vi "Swap_Joysticks.vi"(5 "Hold Time(ms)":u32, 6 "Axes 1 In":T1, 7 "Joystick 1":T2, 8 "Axes 0 in":T1, 9 "Joystick 0":T2) -> (0 "Axes 1 out":T1, 1 "Joystick 1 out":T2, 2 "Axes 0 out":T1, 3 "Joystick 0 Out":T2, 4 "Swap?":bool)   [LabVIEW 2017]
uses:
  ArgosLib/Signal Processing/TypeDefs/EdgeDetector_Type.ctl
  ArgosLib/ArgosLib.lvlib
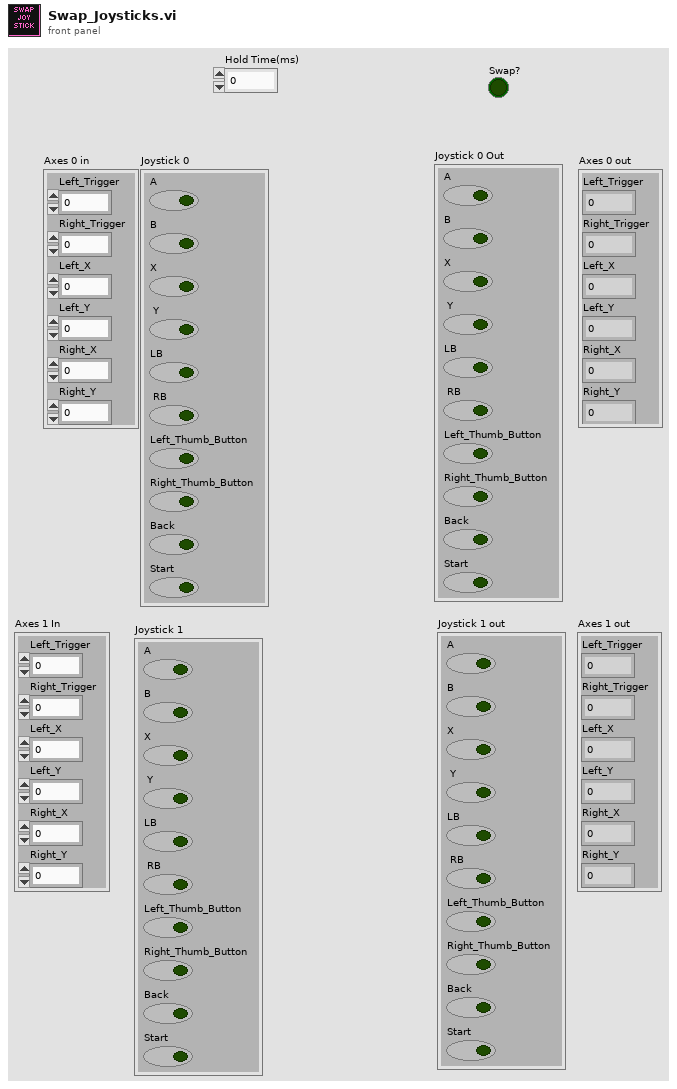
[diagram p1: front panel]
types:
  T1 = cluster{"Left_Trigger":dbl, "Right_Trigger ":dbl, "Left_X":dbl, "Left_Y":dbl, "Right_X":dbl, "Right_Y":dbl}
  T2 = cluster{"A":bool, "B":bool, "X":bool, " Y":bool, "LB":bool, " RB":bool, "Left_Thumb_Button":bool, "Right_Thumb_Button":bool, "Back":bool, "Start":bool}
  T3 = typedef "ArgosLib.lvlib/EdgeDetector_Type.ctl" = enum16{"RisingEdge", "FallingEdge", "Both"}
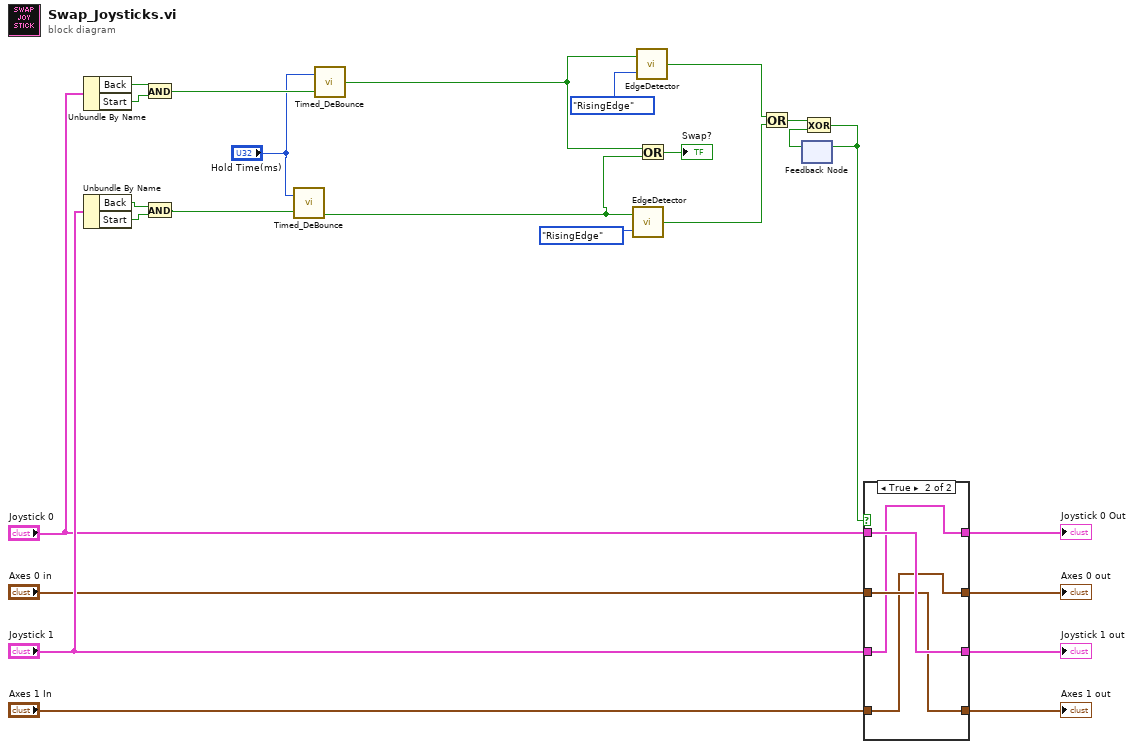
[diagram p0: block diagram]
diagram:
  n1 = Unbundle By Name("Joystick 0") -> ("Back"=w23:bool, "Start"=w22:bool)
  n2 = Unbundle By Name("Joystick 1") -> ("Back"=w25:bool, "Start"=w24:bool)
  n3 = And(x=w23, y=w22) -> (x .and. y?=w3:bool)
  n4 = And(x=w25, y=w24) -> (x .and. y?=w2:bool)
  n5 = call "Timed_DeBounce.vi"("Input"=w2, "Hold Time(ms)"="Hold Time(ms)") -> ("Output"=w5:bool)
  n6 = call "Timed_DeBounce.vi"("Input"=w3, "Hold Time(ms)"="Hold Time(ms)") -> ("Output"=w4:bool)
  n7 = call "EdgeDetector.vi"("DetectorType"=EdgeDetector_Type."RisingEdge", "Input"=w5) -> ("Edge"=w7:bool)
  n8 = call "EdgeDetector.vi"("DetectorType"=EdgeDetector_Type."RisingEdge", "Input"=w4) -> ("Edge"=w12:bool)
  n9 = Or(x=w4, y=w5) -> (x .or. y?=→"Swap?":bool)
  n10 = Or(x=w12, y=w7) -> (x .or. y?=w11:bool)
  n11 = feedback #1() -> (w10:bool)  [unwired: 1 in]
  n12 = Exclusive Or(1:w10, 2:w11) -> (0:w9:bool)
  n13 = feedback-in #1(w9) -> ()
  n14 = case shown="True" w9 {
    tunnel: "Joystick 1" -> [w27 w30]
    tunnel: "Joystick 0" -> [w29 w33]
    tunnel: "Axes 0 in" -> [w28 w32]
    tunnel: "Axes 1 In" -> [w26 w31]
    tunnel: [w29 w30] -> w16
    tunnel: [w28 w31] -> w15
    tunnel: [w27 w33] -> w14
    tunnel: [w26 w32] -> w13
    frame False {
    }
    frame True {
    }
  }
  "Joystick 0 Out" <- w16
  "Axes 0 out" <- w15
  "Joystick 1 out" <- w14
  "Axes 1 out" <- w13
